vi "Pre Launch Init.vi"(11 "ModelCountsObservations in":refnum<class "ModelTimesNObservations.lvclass">) -> (0 "error out":errorcluster, 3 "ModelCountsObservations out":refnum<class "ModelTimesNObservations.lvclass">)   [LabVIEW 2020, in "BenchmarkObservationRate.lvlib" / "ModelTimesNObservations.lvclass"]
doc: "(<B>Filename</B>: Actor Framework.lvlib:Actor.lvclass:Pre Launch Init.vi)\n\nDefines behavior that occurs after the Launch Nested Actor method is invoked but before the actor's Actor Core method begins running.\n\nBy default, this method does nothing. A descendant class may override it to define behavior."
uses:
  ModelTimesNObservations.lvclass
  ModelTimesNObservations.lvclass/ModelTimesNObservations.ctl
  Source/IObserver/IObserver/IObserver.lvclass
  Source/IModel/IModel/IModel.lvclass
  C:/Git/mva-core/Source/IModel/IModel/IModel.lvclass
  C:/Git/mva-core/Source/IObserver/IObserver/IObserver.lvclass
  C:/Program Files (x86)/National Instruments/LabVIEW 2020/vi.lib/ActorFramework/Actor/Actor.lvclass
  C:/Git/mva-core/Test/BechmarkObservationRate/Doubles/ModelCountsObservations/ModelTimesNObservations.lvclass
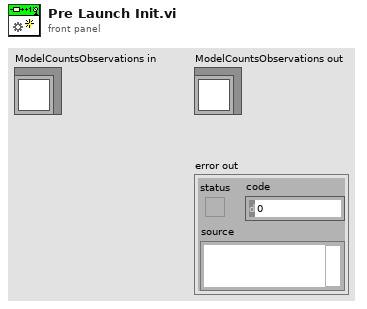
[diagram p1: front panel]
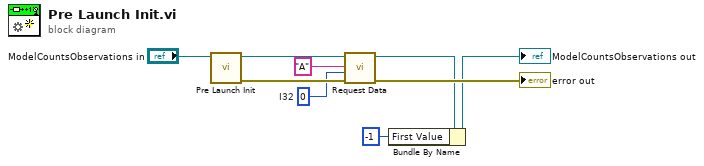
[diagram p0: block diagram]
diagram:
  w3 = 0  # I32
  n1 = call-parent "Pre Launch Init.vi"("IModel in"="ModelCountsObservations in") -> ("error out"=w9:errorcluster, "IModel out"=w6:refnum<class "ModelTimesNObservations.lvclass">)  [unwired: 9 in]
  n2 = call "Request Data.vi"("error in (no error)"=w9, "Data Type"=w3, "Datum Name"="A", "IObserver in"=w6) -> ("error out"=→"error out":errorcluster, "IObserver out"=w5:refnum<class "ModelTimesNObservations.lvclass">)  [unwired: 5 in, 1 out]
  n3 = Bundle By Name(cluster=w5, "First Value"=-1) -> (→"ModelCountsObservations out":refnum<class "ModelTimesNObservations.lvclass">)
